vi "Image_Detect_Object.vi"(6 "Camera":T5=enum."Camera 2", 9 "Detect Crop":bool, 10 "Image Pixels (U32)":u32[][](array[numeric])=array980x440[431200 elements], 11 "Data":T1={"L16 Linear Actuator"="", "XE 1000 Pump"="", "Camera1"="", "Camera2"="", "Camera1_IMG"=refnum, "Camera2_IMG"=refnum, "Img_Capt"=FALSE, "Actuator"=FALSE, "Pump"=FALSE, "Cam 1"=FALSE, "Cam 2"=FALSE, "Empty_Refill"=FALSE, "Crop"=FALSE, "Light intensity"=100, "Exposure Time"=1000.0, "Sample Name"="Test Sample", "Operator"="MRJ", "Calibration 1"=path "C:/Users/au540322/Desktop/IHS_Project/images/Debris/Debris_0/Debris_0_2019_06_01-23-32-49-686.PNG", "Calibration 2"=path "C:/Users/au540322/Desktop/IHS_Project/images/Debris/Debris_0/Debris_0_2019_06_01-23-32-49-686.PNG", "Framerate"=1, "Timeout Sample"=0, "Collection date"="MRJ", "Sample size threshold"=1, "Empty start"=1, "Command"="MRJ", "Calibration Image 1"=refnum, "Calibration Image 2"=refnum, "Original Image 1"=refnum, "Original Image 2"=refnum, "Processing Image 1"=refnum, "Processing Image 2"=refnum, "Object Image 1"=refnum, "Object Image 2"=refnum, "Cam 1 - save queue"=refnum, "Cam 2 - save queue"=refnum, "Station"="", "Species Name"="", "Other Notes"="", "Aperture"=enum."Item 0", "Image Process Queue Size"=500, "Image Save Queue Size"=500, "Overload threshold"=500, "Max Framerate"=100, "Blue Plane Image"=refnum, "Subtract Image"=refnum, "Binary Image 1"=refnum, "ROI mask allocation"=refnum, "Rectangle 1"={"Left"=0, "Top"=0, "Right"=0, "Bottom"=0, "Rotation"=0.0}, "Rectangle 2"={"Left"=0, "Top"=0, "Right"=0, "Bottom"=0, "Rotation"=0.0}, "Binary Image 2"=refnum, "Detection Region %"=0.0, "Cam 1 queue"=refnum, "Cam 2 queue"=refnum, "Detect image 1"=refnum, "Detect image 2"=refnum, "Detect 1"=path "C:/Users/au540322/Desktop/IHS_Project/images/Debris/Debris_0/Debris_0_2019_06_01-23-32-49-686.PNG", "Detect 2"=path "C:/Users/au540322/Desktop/IHS_Project/images/Debris/Debris_0/Debris_0_2019_06_01-23-32-49-686.PNG", "Max large object threshold"=0, "Open(T)/Close(F)"=FALSE} {"Rectangle 2"."Rotation" format="%.2f"; "Rectangle 2"."Left" scale=0.0..1024.0; "Rectangle 2"."Right" scale=0.0..1024.0; "Rectangle 1"."Rotation" format="%.2f"; "Rectangle 1"."Left" scale=0.0..1024.0; "Rectangle 1"."Right" scale=0.0..1024.0; "Max Framerate" min=1; "Overload threshold" min=1; "Image Save Queue Size" min=1; "Image Process Queue Size" min=1; "Empty start" min=1; "Sample size threshold" min=1; "Framerate" min=1; "Light intensity" scale=0.0..100.0}) -> (0 "Object accepted":bool, 1 "Image Binary":T3(plugin-control), 2 "New image":T3(plugin-control), 3 "Crop Image Out":T3(plugin-control), 5 "Object":bool)   [LabVIEW 2019]
uses:
  Camera_ID.ctl
  controls/Data.ctl
  <vilib>/userdefined/High Color/IMAQdx.ctl
  <vilib>/vision/Image Controls.llb/IMAQ Image.ctl
  <vilib>/vision/NI_Vision_Development_Module.lvlib
panel:
  out "x-y":u32
  in  "error in":errorcluster
  out "error out":errorcluster
  in  "Threshold":cluster{"Lower value":sgl, "Upper value":sgl}={"Lower value"=15.0, "Upper value"=255.0} {"Upper value" format="%.2f"; "Lower value" format="%.2f"}
  out "Calibration image in":T3(plugin-control)
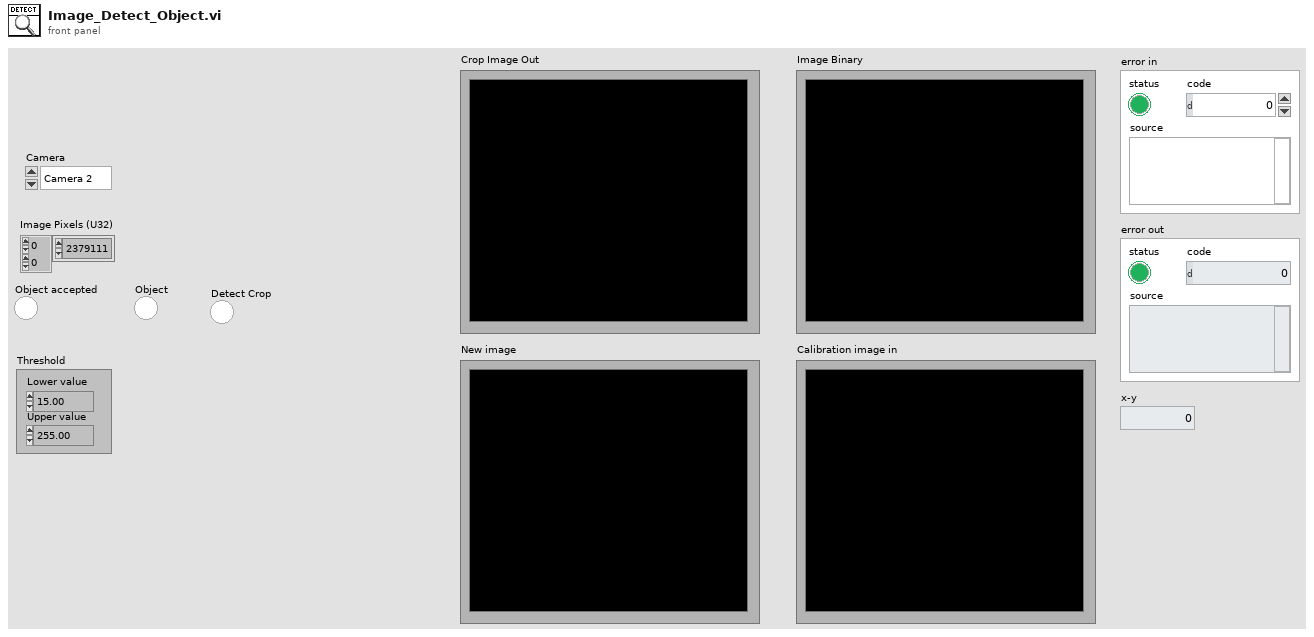
[diagram p1: front panel]
types:
  T1 = typedef "Data.ctl" = cluster{"L16 Linear Actuator":refnum<visa-resource-name>, "XE 1000 Pump":refnum<visa-resource-name>, "Camera1":T2, "Camera2":T2, "Camera1_IMG":T3, "Camera2_IMG":T3, "Img_Capt":bool, "Actuator":bool, "Pump":bool, "Cam 1":bool, "Cam 2":bool, "Empty_Refill":bool, "Crop":bool, "Light intensity":i32, "Exposure Time":dbl, "Sample Name":string, "Operator":string, "Calibration 1":path, "Calibration 2":path, "Framerate":i32, "Timeout Sample":i32, "Collection date":string, "Sample size threshold":i32, "Empty start":u32, "Command":string, "Calibration Image 1":T3, "Calibration Image 2":T3, "Original Image 1":T3, "Original Image 2":T3, "Processing Image 1":T3, "Processing Image 2":T3, "Object Image 1":T3, "Object Image 2":T3, "Cam 1 - save queue":refnum<queue>, "Cam 2 - save queue":refnum<queue>, "Station":string, "Species Name":string, "Other Notes":string, "Aperture":enum32{"Item 0", "Item 1", "Item 2", "Item 3"}, "Image Process Queue Size":i32, "Image Save Queue Size":i32, "Overload threshold":i32, "Max Framerate":i32, "Blue Plane Image":T3, "Subtract Image":T3, "Binary Image 1":T3, "ROI mask allocation":T3, "Rectangle 1":T4, "Rectangle 2":T4, "Binary Image 2":T3, "Detection Region %":dbl, "Cam 1 queue":refnum<queue>, "Cam 2 queue":refnum<queue>, "Detect image 1":T3, "Detect image 2":T3, "Detect 1":path, "Detect 2":path, "Max large object threshold":i32, "Open(T)/Close(F)":bool}
  T2 = typedef "IMAQdx.ctl" = refnum<k21>
  T3 = typedef "IMAQ Image.ctl" = refnum<image>
  T4 = typedef "IMAQ Rectangle" = cluster{"Left":i32, "Top":i32, "Right":i32, "Bottom":i32, "Rotation":dbl}
  T5 = typedef "Camera_ID.ctl" = enum16{"Camera 1", "Camera 2"}
  T6 = cluster{"Global Rectangle":i32[], "Contours":cluster{"ID":enum32{"External", "Internal"}, "Type":u32, "Coordinates":i32[]}[]}
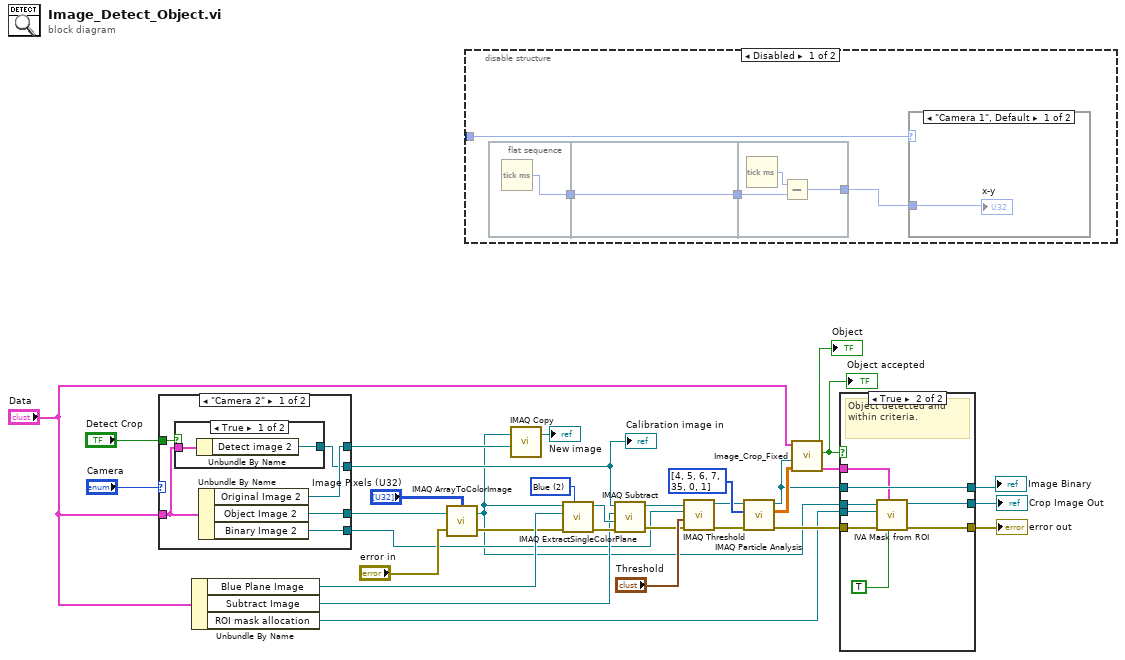
[diagram p0: block diagram]
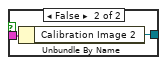
[diagram p4: hidden frame]
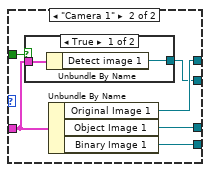
[diagram p5: hidden frame]
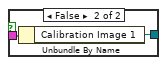
[diagram p6: hidden frame]
diagram:
  w25 = 2 items=["Red", "Green", "Blue", "Hue", "Saturation", "Luminance", "Value", "Intensity"] ("Color Plane")
  w33 = i32[] [4, 5, 6, 7, 35, 0, 1] items=["Center of Mass X", "Center of Mass Y", "First Pixel X", "First Pixel Y", "Bounding Rect Left", "Bounding Rect Top", "Bounding Rect Right", "Bounding Rect Bottom", "Max Feret Diameter Start X", "Max Feret Diameter Start Y", "Max Feret Diameter End X", "Max Feret Diameter End Y", "Max Horiz. Segment Length Left", "Max Horiz. Segment Length Right", "Max Horiz. Segment Length Row", "-", "Bounding Rect Width", "Bounding Rect Height", "Bounding Rect Diagonal", "Perimeter", "Convex Hull Perimeter", "Holes' Perimeter", "Max Feret Diameter", "Equivalent Ellipse Major Axis", "Equivalent Ellipse Minor Axis", "Equivalent Ellipse Minor Axis (Feret)", "Equivalent Rect Long Side", "Equivalent Rect Short Side", "Equivalent Rect Diagonal", "Equivalent Rect Short Side (Feret)", "Average Horiz. Segment Length", "Average Vert. Segment Length", "Hydraulic Radius", "Waddel Disk Diameter", "-", "Area", "Holes' Area", "Particle & Holes' Area", "Convex Hull Area", "Image Area", "-", "Number of Holes", "Number of Horiz. Segments", "Number of Vert. Segments", "-", "Orientation", "Max Feret Diameter Orientation", "-", "% Area/Image Area", "% Area/(Particle & Holes' Area)", "Ratio of Equivalent Ellipse Axes", "Ratio of Equivalent Rect Sides", "-", "Elongation Factor", "Compactness Factor", "Heywood Circularity Factor", "Type Factor", "-", "Sum X", "Sum Y", "Sum XX", "Sum XY", "Sum YY", "Sum XXX", "Sum XXY", "Sum XYY", "Sum YYY", "-", "Moment of Inertia XX", "Moment of Inertia XY", "Moment of Inertia YY", "Moment of Inertia XXX", "Moment of Inertia XXY", "Moment of Inertia XYY", "Moment of Inertia YYY", "Norm. Moment of Inertia XX", "Norm. Moment of Inertia XY", "Norm. Moment of Inertia YY", "Norm. Moment of Inertia XXX", "Norm. Moment of Inertia XXY", "Norm. Moment of Inertia XYY", "Norm. Moment of Inertia YYY", "Hu Moment 1", "Hu Moment 2", "Hu Moment 3", "Hu Moment 4", "Hu Moment 5", "Hu Moment 6", "Hu Moment 7"] ("Pixel Measurements")
  n1 = case shown="\"Camera 2\"" "Camera" {
    tunnel: "Data" -> [w35 w45]
    tunnel: [w34 w46] -> w15
    tunnel: [w39 w49] -> w14
    tunnel: [w38 w48] -> w9
    tunnel: [w37 w47] -> w6
    tunnel: "Detect Crop" -> [w36 w44]
    frame "Camera 2" {
      n2 = case shown="True" w36 {
        tunnel: w35 -> [w41 w43]
        tunnel: [w40 w42] -> w34
        frame True {
          n3 = Unbundle By Name(w41) -> ("Detect image 2"=w40:T3)
        }
        frame False {
          n4 = Unbundle By Name(w43) -> ("Calibration Image 2"=w42:T3)
        }
      }
      n5 = Unbundle By Name(w35) -> ("Original Image 2"=w38:T3, "Object Image 2"=w39:T3, "Binary Image 2"=w37:T3)
    }
    frame "Camera 1" {
      n6 = case shown="True" w44 {
        tunnel: w45 -> [w51 w53]
        tunnel: [w50 w52] -> w46
        frame True {
          n7 = Unbundle By Name(w51) -> ("Detect image 1"=w50:T3)
        }
        frame False {
          n8 = Unbundle By Name(w53) -> ("Calibration Image 1"=w52:T3)
        }
      }
      n9 = Unbundle By Name(w45) -> ("Original Image 1"=w48:T3, "Object Image 1"=w49:T3, "Binary Image 1"=w47:T3)
    }
  }
  "Calibration image in" <- w15
  n10 = Unbundle By Name("Data") -> ("Blue Plane Image"=w12:T3, "Subtract Image"=w11:T3, "ROI mask allocation"=w7:T3)
  n11 = call "IMAQ ArrayToColorImage"("Image Pixels (U32)"="Image Pixels (U32)", "Image"=w14, "error in (no error)"="error in") -> ("Image Out"=w1:T3, "error out"=w2:errorcluster)  [unwired: 2 in]
  n12 = disable-structure shown="Disabled" {
    disable-tunnel: _ -> [w54 _]
    frame Disabled {
      n13 = flat-sequence {
        tunnel: [w59] -> w57
        tunnel: w57 -> [w60]
        tunnel: [w60] -> w56
        tunnel: w56 -> [w62]
        tunnel: [w61] -> w55
        frame #0 {
          n14 = Tick Count (ms)() -> (millisecond timer value=w59:u32)
        }
        frame #1 {
        }
        frame #2 {
          n15 = Tick Count (ms)() -> (millisecond timer value=w63:u32)
          n16 = Subtract(x=w63, y=w62) -> (x-y=w61:u32)
        }
      }
      n17 = case shown="\"Camera 1\", Default" w54 {
        tunnel: w55 -> [w58 _]
        frame "Camera 1", Default {
          "x-y" <- w58
        }
        frame "Camera 2" {
        }
      }
    }
    frame Enabled {
    }
  }
  n18 = call "IMAQ Copy"("Image Dst"=w9, "Image Src"=w1) -> ("Image Dst Out"=→"New image":T3)  [unwired: 4 in, 1 out]
  n19 = call "IMAQ ExtractSingleColorPlane"("Color Plane"=w25, "error in (no error)"=w2, "Image Dst"=w12, "Image Src"=w1) -> ("error out"=w18:errorcluster, "Image Dst Out"=w19:T3)  [unwired: 6 out]
  n20 = call "IMAQ Subtract"("Image Src A"=w15, "Image Dst"=w11, "Image Src B"=w19, "error in (no error)"=w18) -> ("Image Dst Out"=w16:T3, "error out"=w17:errorcluster)  [unwired: 1 in, 2 out]
  n21 = call "IMAQ Threshold"("error in (no error)"=w17, "Range"="Threshold", "Image Dst"=w6, "Image Src"=w16) -> ("error out"=w22:errorcluster, "Image Dst Out"=w24:T3)  [unwired: 2 in, 4 out]
  n22 = call "IMAQ Particle Analysis"("error in (no error)"=w22, "Pixel Measurements"=w33, "Image"=w24) -> ("error out"=w26:errorcluster, "Particle Measurements (Pixels)"=w32:dbl[][], "Image Out (duplicate)"=w29:T3)  [unwired: 2 in, 4 out]
  n23 = call "Image_Crop_Fixed.vi"("Particle Measurements"=w32, "Image  in"=w29, "Data"="Data") -> ("ROI descriptor"=w31:T6, "Object accept"=w5:bool, "Object"=→"Object":bool)  [unwired: 6 in]
  "Object accepted" <- w5
  n24 = case shown="True" w5 {
    tunnel: [w64 w73] -> w27
    tunnel: w26 -> [w65 w69]
    tunnel: [w66 w72] -> w28
    tunnel: w29 -> [w66 w72]
    tunnel: [w65 w68] -> w21
    tunnel: w31 -> [_ w71]
    tunnel: w7 -> [_ w70]
    tunnel: w1 -> [w64 w67]
    frame False {
      # "No object found or not within criteria."
    }
    frame True {
      # "Object detected and within criteria."
      n25 = call <vilib>:"IVA Mask from ROI.vi"("Shrink"=TRUE, "ROI Descriptor"=w71, "error in (no error)"=w69, "Mask allocation"=w70, "Image Src"=w67) -> ("error out"=w68:errorcluster, "Image Out"=w73:T3)  [unwired: 1 in, 4 out]
    }
  }
  "Crop Image Out" <- w27
  "Image Binary" <- w28
  "error out" <- w21
